vi "생산자_소비자 실습.vi"() -> ()   [LabVIEW 2020]
panel:
  out "추가된 배열":enum16{"초기화", "측정", "정지", "일시정지"}[](array[ring])
  in  "일시정지":bool
  out "웨이브폼 차트":dbl(graph)
  in  "정지":bool
  in  "측정":bool
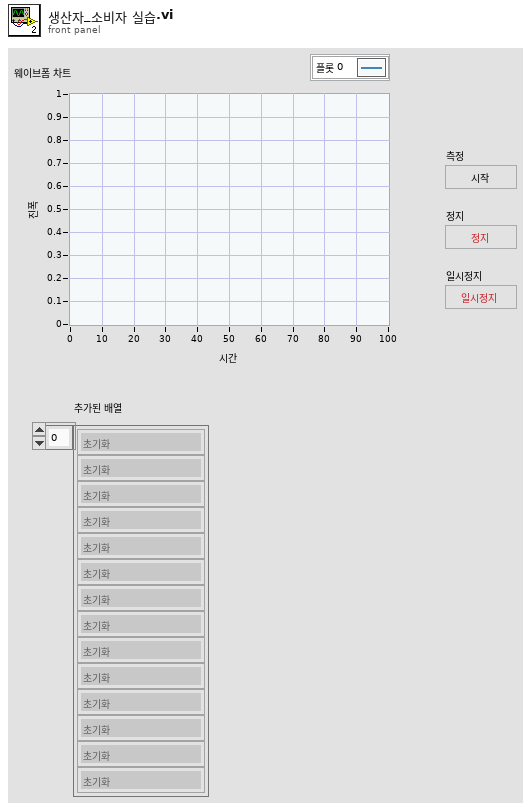
[diagram p1: front panel]
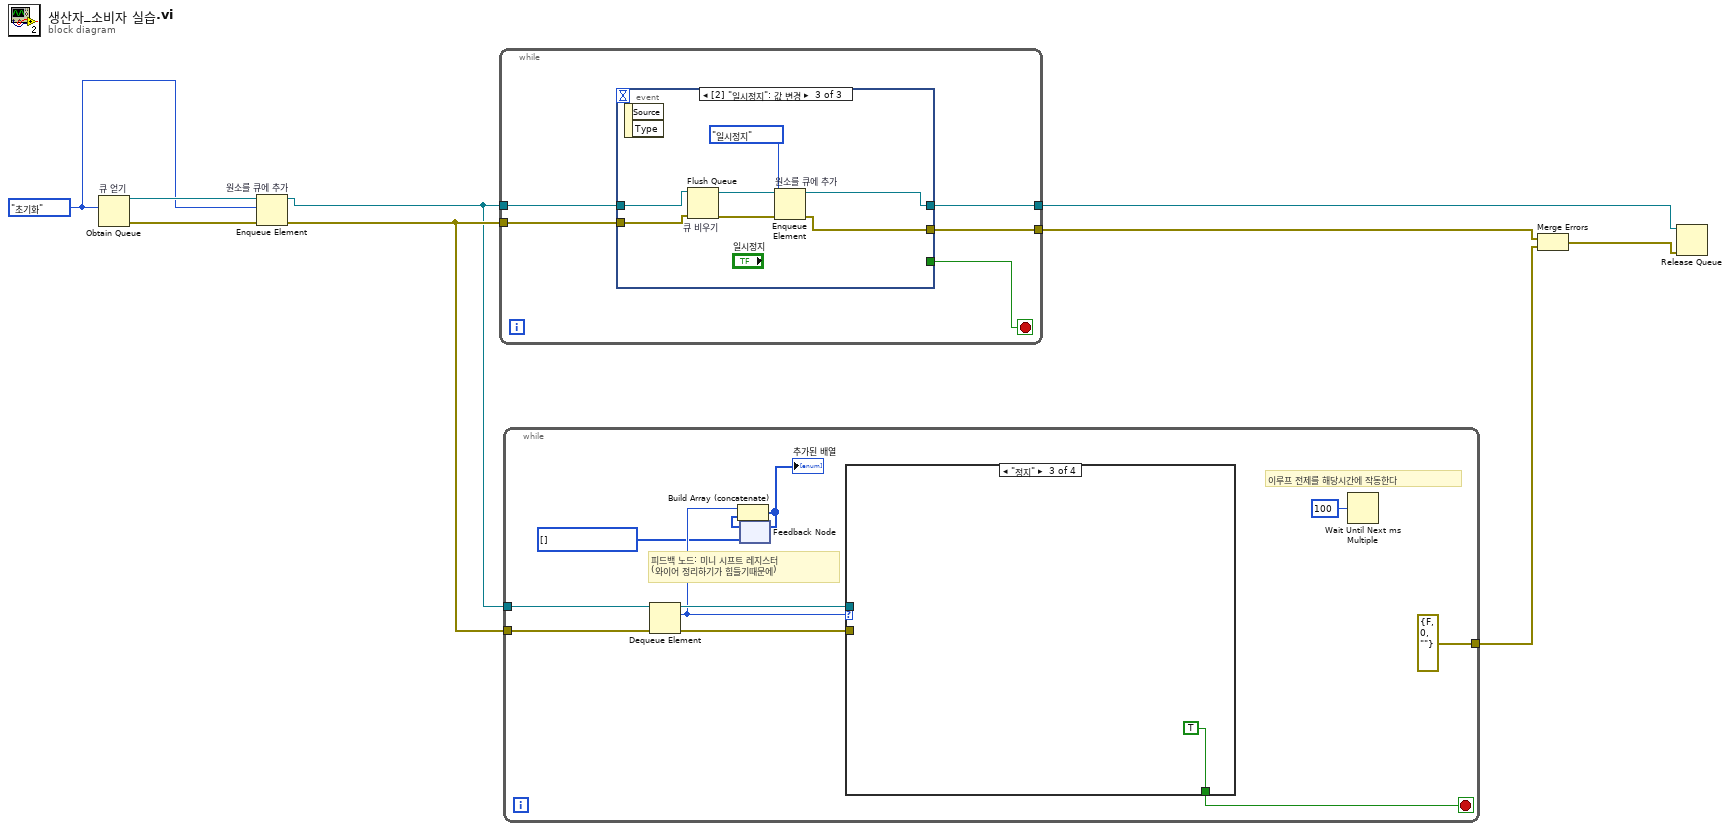
[diagram p0: block diagram]
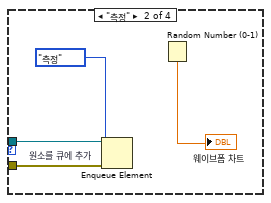
[diagram p3: hidden frame]
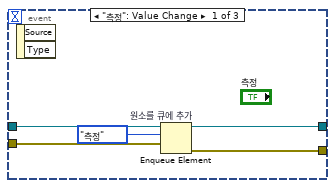
[diagram p5: hidden frame]
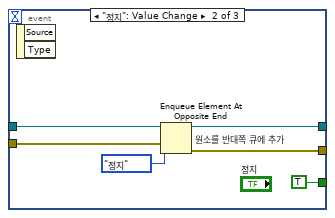
[diagram p6: hidden frame]
diagram:
  w1 = enum16{"초기화", "측정", "정지", "일시정지"}."초기화"
  n1 = Obtain Queue "큐 얻기"(element data type=w1) -> (queue out=w2:refnum<queue>, error out=w5:errorcluster)  [unwired: 4 in, 1 out]
  n2 = Enqueue Element "원소를 큐에 추가"(queue=w2, element=w1, error in (no error)=w5) -> (queue out=w3:refnum<queue>, error out=w4:errorcluster)  [unwired: 1 in, 1 out]
  n3 = while {
    tunnel: w3 -> [w14]
    tunnel: w4 -> [w13]
    tunnel: [w12] -> w9
    tunnel: [w11] -> w6
    stop <- w10 stop-if-true
    n4 = event shown="[2] \"일시정지\": 값 변경" {
      selector: _ -> [_ _ _]
      dyn-events: _ -> [_ _ _]
      timeout: _ -> [_ _ _]
      tunnel: w14 -> [w19 w25 w32]
      tunnel: w13 -> [w18 w24 w31]
      tunnel: [w17 w23 w28] -> w12
      tunnel: [w16 w22 w27] -> w11
      tunnel: [_ TRUE _] -> w10
      event "측정": Value Change {
        n5 = event-data() -> ()  [unwired: 1 in, 2 out]
        n6 = Enqueue Element "원소를 큐에 추가"(queue=w19, element=enum16{"초기화", "측정", "정지", "일시정지"}."측정" ("원소"), error in (no error)=w18) -> (queue out=w16:refnum<queue>, error out=w17:errorcluster)  [unwired: 1 in, 1 out]
      }
      event "정지": Value Change {
        n7 = event-data() -> ()  [unwired: 1 in, 2 out]
        n8 = Enqueue Element At Opposite End "원소를 반대쪽 큐에 추가"(queue=w25, element=enum16{"초기화", "측정", "정지", "일시정지"}."정지" ("원소"), error in (no error)=w24) -> (queue out=w22:refnum<queue>, error out=w23:errorcluster)  [unwired: 1 in, 1 out]
      }
      event "일시정지": Value Change {
        n9 = event-data() -> ()  [unwired: 1 in, 2 out]
        n10 = Flush Queue "큐 비우기"(queue=w32, error in (no error)=w31) -> (queue out=w30:refnum<queue>, error out=w29:errorcluster)  [unwired: 1 out]
        n11 = Enqueue Element "원소를 큐에 추가"(queue=w30, element=enum16{"초기화", "측정", "정지", "일시정지"}."일시정지" ("원소"), error in (no error)=w29) -> (queue out=w27:refnum<queue>, error out=w28:errorcluster)  [unwired: 1 in, 1 out]
      }
    }
  }
  n12 = while {
    tunnel: w3 -> [w43]
    tunnel: w4 -> [w42]
    tunnel: [errorcluster {"status"=FALSE, "code"=0, "source"=""} ("에러 상수")] -> w8
    stop <- w40 stop-if-true
    w33 = enum16{"초기화", "측정", "정지", "일시정지"}[] [] items=["초기화", "측정", "정지", "일시정지"]
    # "피드백 노드: 미니 시프트 레지스터\n(와이어 정리하기가 힘들기때문에)"
    # "이루프 전제를 해당시간에 작동한다"
    n13 = Dequeue Element(queue=w43, error in (no error)=w42) -> (queue out=w39:refnum<queue>, element=w36:enum16{"초기화", "측정", "정지", "일시정지"}, error out=w38:errorcluster)  [unwired: 1 in, 1 out]
    n14 = feedback #1(w33) -> (w34:enum16{"초기화", "측정", "정지", "일시정지"}[])
    n15 = Build Array (concatenate)(w36, w34) -> (w35:enum16{"초기화", "측정", "정지", "일시정지"}[])
    "추가된 배열" <- w35
    n16 = feedback-in #1(w35) -> ()
    n17 = case shown="\"정지\"" w36 {
      tunnel: [_ _ TRUE _] -> w40
      tunnel: w39 -> [_ w46 _ _]
      tunnel: w38 -> [_ w45 _ _]
      frame "초기화", Default {
      }
      frame "측정" {
        n18 = Enqueue Element "원소를 큐에 추가"(queue=w46, element=enum16{"초기화", "측정", "정지", "일시정지"}."측정" ("원소"), error in (no error)=w45) -> ()  [unwired: 1 in, 3 out]
        n19 = Random Number (0-1)() -> (number: 0 to 1=→"웨이브폼 차트":dbl)
      }
      frame "정지" {
      }
      frame "일시정지" {
      }
    }
    n20 = Wait Until Next ms Multiple(millisecond multiple=u32 100 ("ms 배수")) -> ()  [unwired: 1 out]
  }
  n21 = Merge Errors(w9, w8) -> (w7:errorcluster)
  n22 = Release Queue(queue=w6, error in (no error)=w7) -> ()  [unwired: 1 in, 3 out]
